vi "savecluster_V0.01.vi"(11 "Cluster (Eingang)":refnum<vi>) -> ()   [LabVIEW 2014]
uses:
  <vilib>/Utility/xml.llb/Write to XML File(string).vi
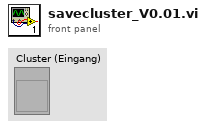
[diagram p1: front panel]
types:
  T1 = cluster{"Fahrzeugdaten":string, "date/time string":string, "Rolle [Inkr/U]":u16, "Rollenumfang [m]":dbl, "Rollenträgheit [kgm²]":dbl, "Zündung [Imp/U]":u8, "Getriebe [1:]":dbl, "Reifenumfang [m] ":dbl, "element":dbl, "Gl. Mittelwert":u8, "Differenzenquotient":u8, "Polynom":u8, "element":dbl, "element":dbl, "Lufttemperatur [°C]":dbl, "Luftfeuchtigkeit [%]":dbl, "Luftdruck [mbar]":dbl, dbl[], dbl[], "Best Polynomial Fit":dbl[], dbl[], "Übersetzung ermitteln aus":u8, "[s]":dbl, "nmin [1/min]":dbl, "nmax [1/min]":dbl, "n vom Gas [1/min]":dbl, dbl[], i32[], "Boolesch":bool}
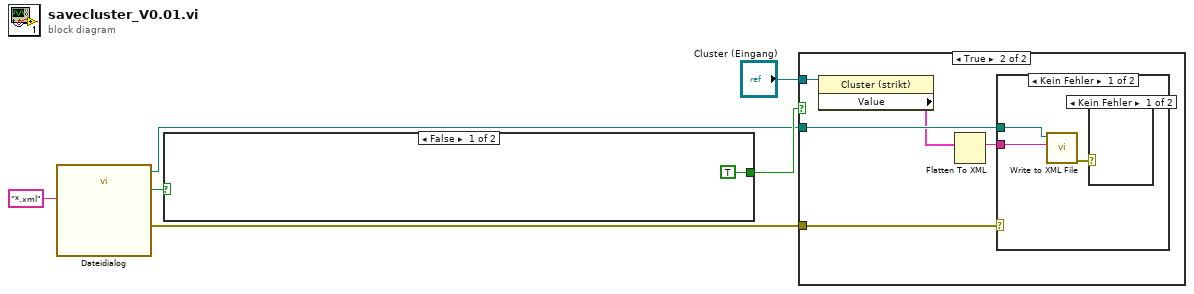
[diagram p0: block diagram]
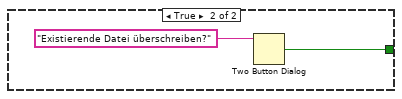
[diagram p5: hidden frame]
diagram:
  n1 = call "Dateidialog"("pattern (all files)"="*.xml") -> ("selected path"=w2:path, "exists"=w5:bool, "error out"=w4:errorcluster)  [unwired: 11 in, 1 out]
  n2 = case shown="False" w5 {
    tunnel: [TRUE ("T button?") w8] -> w6
    frame False {
    }
    frame True {
      n3 = Two Button Dialog(message="Existierende Datei überschreiben?" ("Nachricht")) -> (T button?=w8:bool)  [unwired: 2 in]
    }
  }
  n4 = case shown="True" w6 {
    tunnel: w2 -> [_ w14]
    tunnel: w4 -> [_ w13]
    tunnel: "Cluster (Eingang)" -> [_ w10]
    frame False {
    }
    frame True {
      n5 = property on="Eigenschaftsknoten" class="Cluster (strikt)"(reference=w10) -> ("Value"=w11:T1)  [unwired: 1 in, 2 out]
      n6 = Flatten To XML(anything=w11) -> (xml string=w12:string)
      n7 = case shown="Kein Fehler" w13 {
        tunnel: w12 -> [w17 _]
        tunnel: w14 -> [w15 _]
        frame No Error {
          n8 = call-poly <vilib>:"Write to XML File.vi"("XML Input"=w17, "XML File Path"=w15) -> ("error out"=w16:errorcluster)  [unwired: 7 in, 2 out]
          n9 = case shown="Kein Fehler" w16 {
            frame No Error {
            }
            frame Error {
            }
          }
        }
        frame Error {
        }
      }
    }
  }
